vi "FTW-Context-Destroy.vi"(11 "error in":errorcluster) -> (15 "error out":errorcluster)   [LabVIEW 2013, in "FTW-Actor-Context.lvclass"]
uses:
  FTW-Actor-Context.lvclass
  logger/FTW-Logger.lvclass
  FTW-Context-Instance.vi
panel:
  # "Inputs"
  # "Outputs"
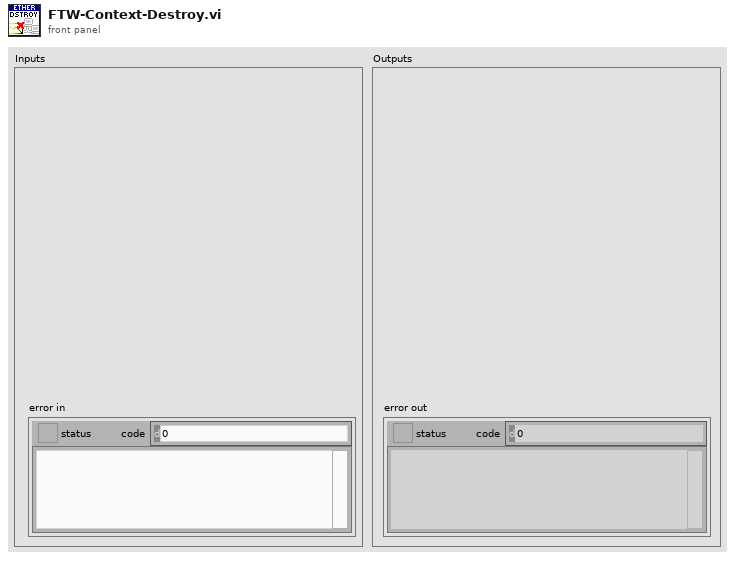
[diagram p1: front panel]
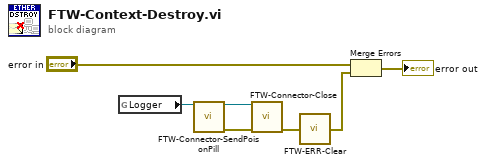
[diagram p0: block diagram]
diagram:
  n1 = global read "FTW-Context-Instance.vi" "Logger"() -> (w1:refnum<class "FTW-Logger.lvclass">)
  n2 = call-dynamic "FTW-Connector-SendPoisonPill.vi"("FTW Actor Connector"=w1) -> ("FTW Actor Connector out"=w5:refnum<class "FTW-Logger.lvclass">, "error out"=w4:errorcluster)  [unwired: 11 in, 2 out]
  n3 = call-dynamic "FTW-Connector-Close.vi"("FTW Actor Connector"=w5, "error in"=w4) -> ("error out"=w2:errorcluster)  [unwired: 13 in]
  n4 = call "FTW-ERR-Clear.vi"("error to snuff"=w2) -> ("no error"=w3:errorcluster)
  n5 = Merge Errors("error in", w3) -> (→"error out":errorcluster)
